vi "get wire mode.vi"(8 "error in (no error)":errorcluster, 11 "Modbus Slave configuration in":refnum<class "Modbus Module configuration.lvclass">) -> (0 "error out":errorcluster, 2 "Wire Mode":i16(ring)=-1 items=["Unknown"=-1, "RS485/Wire4"=0, "RS485/Wire2-EchoDTR"=1, "RS485/Wire2-CtrlDTR"=2, "RS485/Wire2-Auto"=3, "RS232/DTE"=128, "RS232/DCE"=129, "RS232/AUTO"=130], 3 "Modbus Slave configuration out":refnum<class "Modbus Module configuration.lvclass">)   [LabVIEW 2013, in "Modbus Module configuration.lvclass"]
uses:
  Modbus Module configuration.lvclass
  Modbus Module configuration.lvclass/Modbus Module configuration.ctl
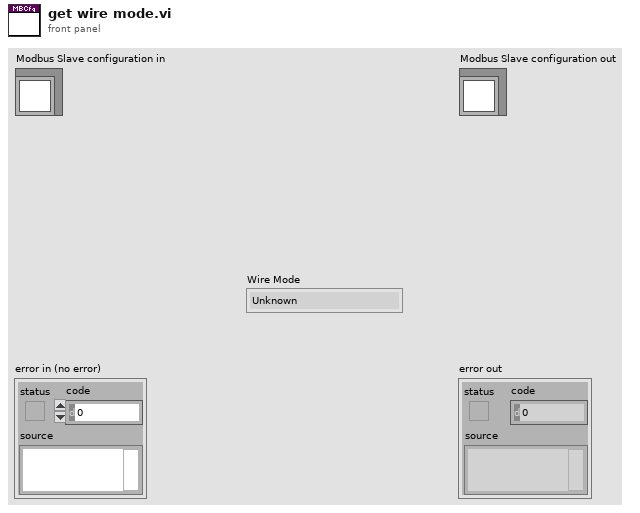
[diagram p1: front panel]
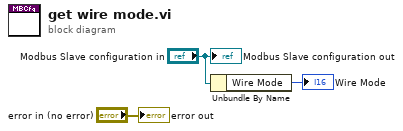
[diagram p0: block diagram]
diagram:
  n1 = Unbundle By Name("Modbus Slave configuration in") -> ("Wire Mode"=→"Wire Mode":i16)
  "error out" <- "error in (no error)"
  "Modbus Slave configuration out" <- "Modbus Slave configuration in"
